vi "get_output_range.vi"(8 "error in (no error)":errorcluster, 10 "Ouptut ranges":string(combo)="0", 11 "VISA Refnum in":refnum<visa-resource-name>) -> (0 "error out":errorcluster, 3 "VISA Refnum out":refnum<visa-resource-name>)   [LabVIEW 2018]
panel:
  out "Output range":string
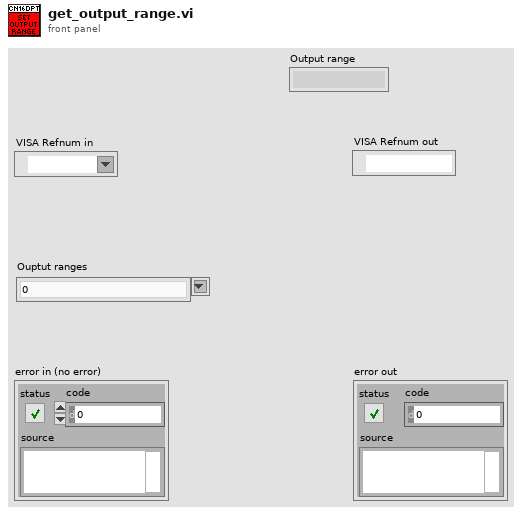
[diagram p1: front panel]
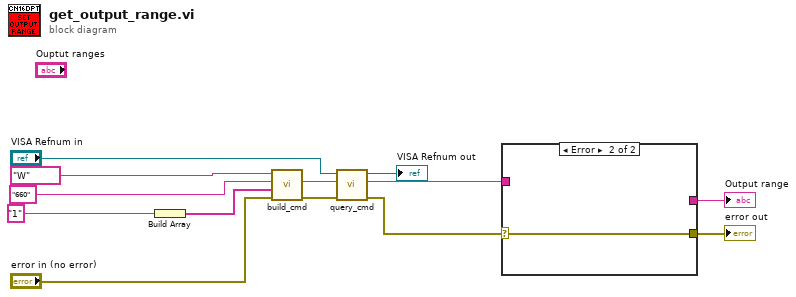
[diagram p0: block diagram]
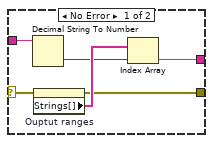
[diagram p2: hidden frame]
diagram:
  n1 = Build Array("1" ("element")) -> (w6:string[])
  n2 = call "build_cmd.vi"("error in (no error)"="error in (no error)", "Parameter list"=w6, "Command ID"="660", "Command class"="W") -> ("error out"=w8:errorcluster, "Command"=w7:string)  [unwired: 6 in]
  n3 = call "query_cmd.vi"("error in (no error)"=w8, "Command"=w7, "VISA resource name"="VISA Refnum in") -> ("error out"=w4:errorcluster, "Response"=w3:string, "VISA resource name out"=→"VISA Refnum out":refnum<visa-resource-name>)  [unwired: 6 in]
  n4 = case shown="Error" w4 {
    selector: w4 -> [w19 w20]
    tunnel: w3 -> [w18 _]
    tunnel: [w15 _] -> w2
    tunnel: [w14 w20] -> w1
    frame No Error {
      n5 = Decimal String To Number(string=w18) -> (number=w16:i32)  [unwired: 2 in, 1 out]
      n6 = property on="Ouptut ranges" class="CmbBox"(error in=w19) -> (error out=w14:errorcluster, "Strings[]"=w17:string[])  [unwired: 1 in, 1 out]
      n7 = Index Array(array=w17, index=w16) -> (element=w15:string)
    }
    frame Error {
    }
  }
  "error out" <- w1
  "Output range" <- w2
